vi "test_PipelineResult_CreateFromPacket.vi"() -> ()   [LabVIEW 2019]
uses:
  PhotonVisionLib/TypeDef/PhotonPipelineResultType.ctl
  PhotonVisionLib/TypeDef/PhotonTrackedTargetType.ctl
  PhotonVisionLib/TypeDef/TargetCornerType.ctl
  <vilib>/Rock Robotics/WPI/ThirdParty/JAS_Junk/TrajLib/TypeDef/TRANSFORM3D.ctl
  <vilib>/Rock Robotics/WPI/ThirdParty/JAS_Junk/TrajLib/TypeDef/TRANSLATION3D.ctl
  <vilib>/Rock Robotics/WPI/ThirdParty/JAS_Junk/TrajLib/TypeDef/ROTATION3D.ctl
  <vilib>/Rock Robotics/WPI/ThirdParty/JAS_Junk/TrajLib/TypeDef/QUATERNION.ctl
  PhotonVisionLib/PhotonVisionLib.lvlib
  <vilib>/Rock Robotics/WPI/ThirdParty/JAS_Junk/TrajLib/Trajectory_Library.lvlib
panel:
  out "PhotonPipelineResult":T1 {"Targets"."AltCameraToTarget"."TRANSLATION3D"."Z" format="%14.3f"; "Targets"."AltCameraToTarget"."TRANSLATION3D"."Y" format="%14.3f"; "Targets"."AltCameraToTarget"."TRANSLATION3D"."X" format="%14.3f"; "Targets"."BestCameraToTarget"."TRANSLATION3D"."Z" format="%14.3f"; "Targets"."BestCameraToTarget"."TRANSLATION3D"."Y" format="%14.3f"; "Targets"."BestCameraToTarget"."TRANSLATION3D"."X" format="%14.3f"}
  in  "RawData":u8[](array[numeric])=[63, 240, 0, 0, 0, 0, 0, 0, 1, 63, 248, 0, 0, 0, 0, 0, 0, 63, 248, 0, 0, 0, 0, 0, 0, 63, 240, 0, 0, 0, 0, 0, 0, 63, 240, 0, 0, 0, 0, 0, 0, 63, 240, 0, 0, 0, 0, 0, 0, 63, 240, 0, 0, 0, 0, 0, 0, 63, 240, 0, 0, 0, 0, 0, 0, 63, 240, 0, 0, 0, 0, 0, 0, 63, 240, 0, 0, 0, 0, 0, 0, 63, 240, 0, 0, 0, 0, 0, 0, 63, 240, 0, 0, 0, 0, 0, 0, 63, 240, 0, 0, 0, 0, 0, 0, 63, 240, 0, 0, 0, 0, 0, 0, 63, 240, 0, 0, 0, 0, 0, 0, 63, 240, 202, 202, 202, 0, 0, 0] format="%x"
  # "OLD -- THIS IS WRONG NOW...\n\nPrefix is 9 bytes\n\nEach Target is 15 x 8 bytes = 120 bytes"
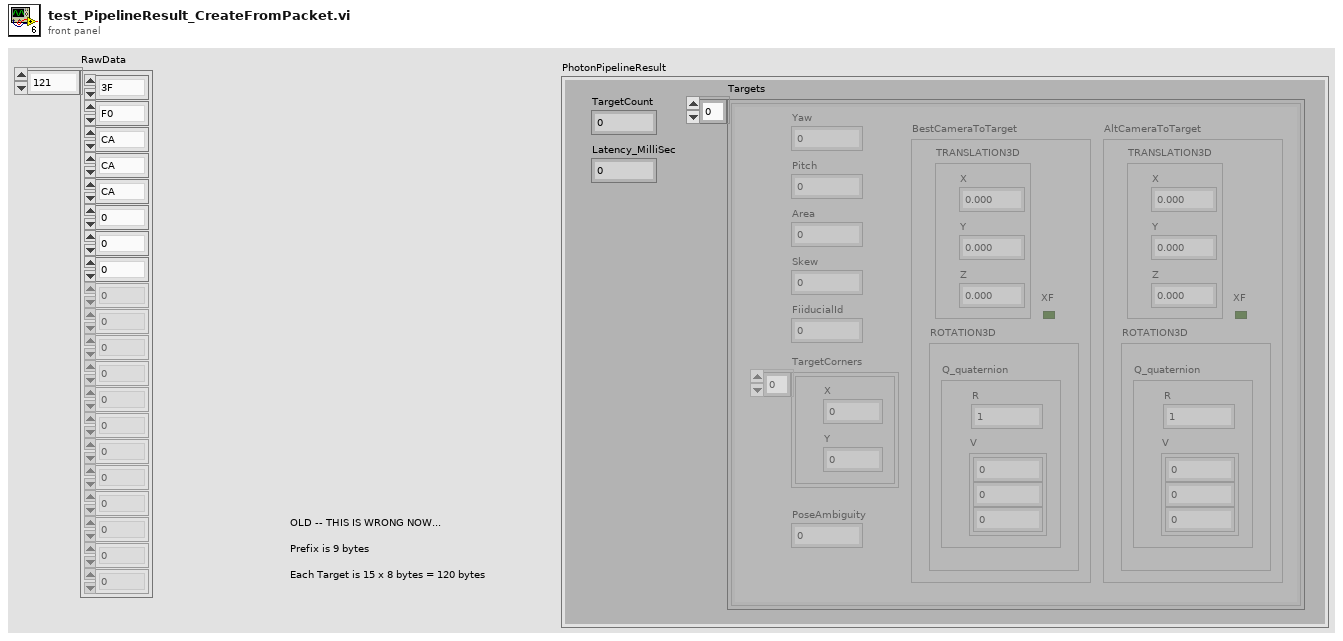
[diagram p1: front panel]
types:
  T1 = typedef "PhotonVisionLib.lvlib/PhotonPipelineResultType.ctl" = cluster{"TargetCount":i32, "Latency_MilliSec":dbl, "Targets":T2[]}
  T2 = typedef "PhotonVisionLib.lvlib/PhotonTrackedTargetType.ctl" = cluster{"Yaw":dbl, "Pitch":dbl, "Area":dbl, "Skew":dbl, "TargetCorners":T3[], "BestCameraToTarget":T4, "FiiducialId":i32, "AltCameraToTarget":T4, "PoseAmbiguity":dbl}
  T3 = typedef "PhotonVisionLib.lvlib/TargetCornerType.ctl" = cluster{"X":dbl, "Y":dbl}
  T4 = typedef "Trajectory_Library.lvlib/TRANSFORM3D.ctl" = cluster{"TRANSLATION3D":T5, "ROTATION3D":T6, "XF":bool}
  T5 = typedef "Trajectory_Library.lvlib/TRANSLATION3D.ctl" = cluster{"X":dbl, "Y":dbl, "Z":dbl}
  T6 = typedef "Trajectory_Library.lvlib/ROTATION3D.ctl" = cluster{"Q_quaternion":T7}
  T7 = typedef "Trajectory_Library.lvlib/QUATERNION.ctl" = cluster{"R":dbl, "V":dbl[]}
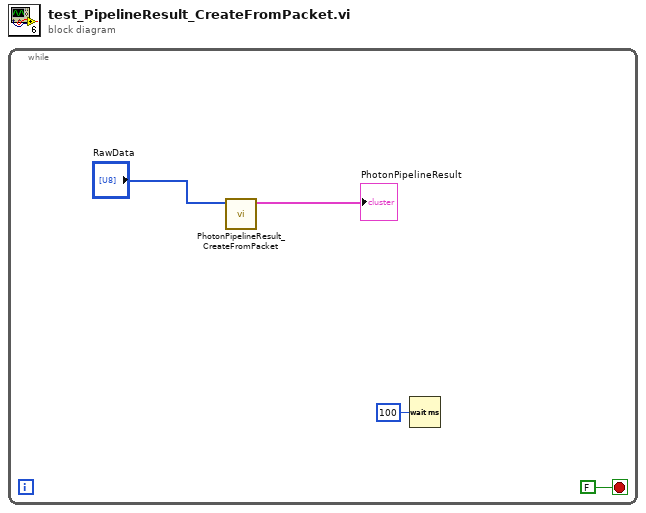
[diagram p0: block diagram]
diagram:
  n1 = while {
    stop <- FALSE stop-if-true
    n2 = call "PhotonPipelineResult_CreateFromPacket.vi"("RawData"="RawData") -> ("PhotonPipelineResult"=→"PhotonPipelineResult":T1)  [unwired: 10 in]
    n3 = Wait (ms)(milliseconds to wait=u32 100) -> ()  [unwired: 1 out]
  }
